vi "Build Tree.vi"(5 "Panel":refnum<vi>, 7 "Tree":refnum<vi>, 9 "Changed Actors":refnum<class "Message Enqueuer.lvclass">[](array[class]), 10 "Monitor Data":refnum<class "Monitor Data.lvclass">) -> (2 "Stopped Actors":string[](array[string]))   [LabVIEW 2023, in "Monitored Actor.lvlib" / "Classic Monitor.lvclass"]
doc: "Manages the tree.\n\nCopyright: MGI 2016\nAuthor: Derek Trepanier"
uses:
  Classic Monitor.lvclass
  Monitor Data/Monitor Data.lvclass
  builds/Framework/Actor Framework.lvlibp/1abvi3w/vi.lib/ActorFramework/Message Enqueuer/Message Enqueuer.lvclass
  Classic Monitor.lvclass/Classic Monitor.ctl
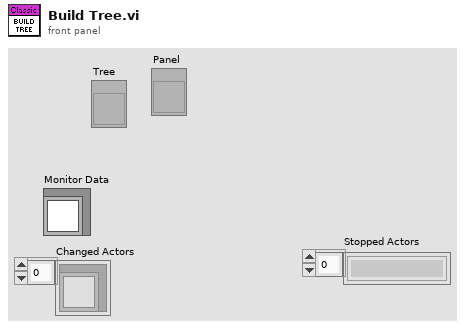
[diagram p1: front panel]
types:
  T1 = typedef "Monitored Actor.lvlib/Monitor Data.lvclass/Actor Data.ctl" = cluster{"Actor Type":string, "Actor Core VI":string, "Self":refnum<class "Message Enqueuer.lvclass">, "Caller":refnum<class "Message Enqueuer.lvclass">, "Actor Label":string, "Last Ping":dbl}
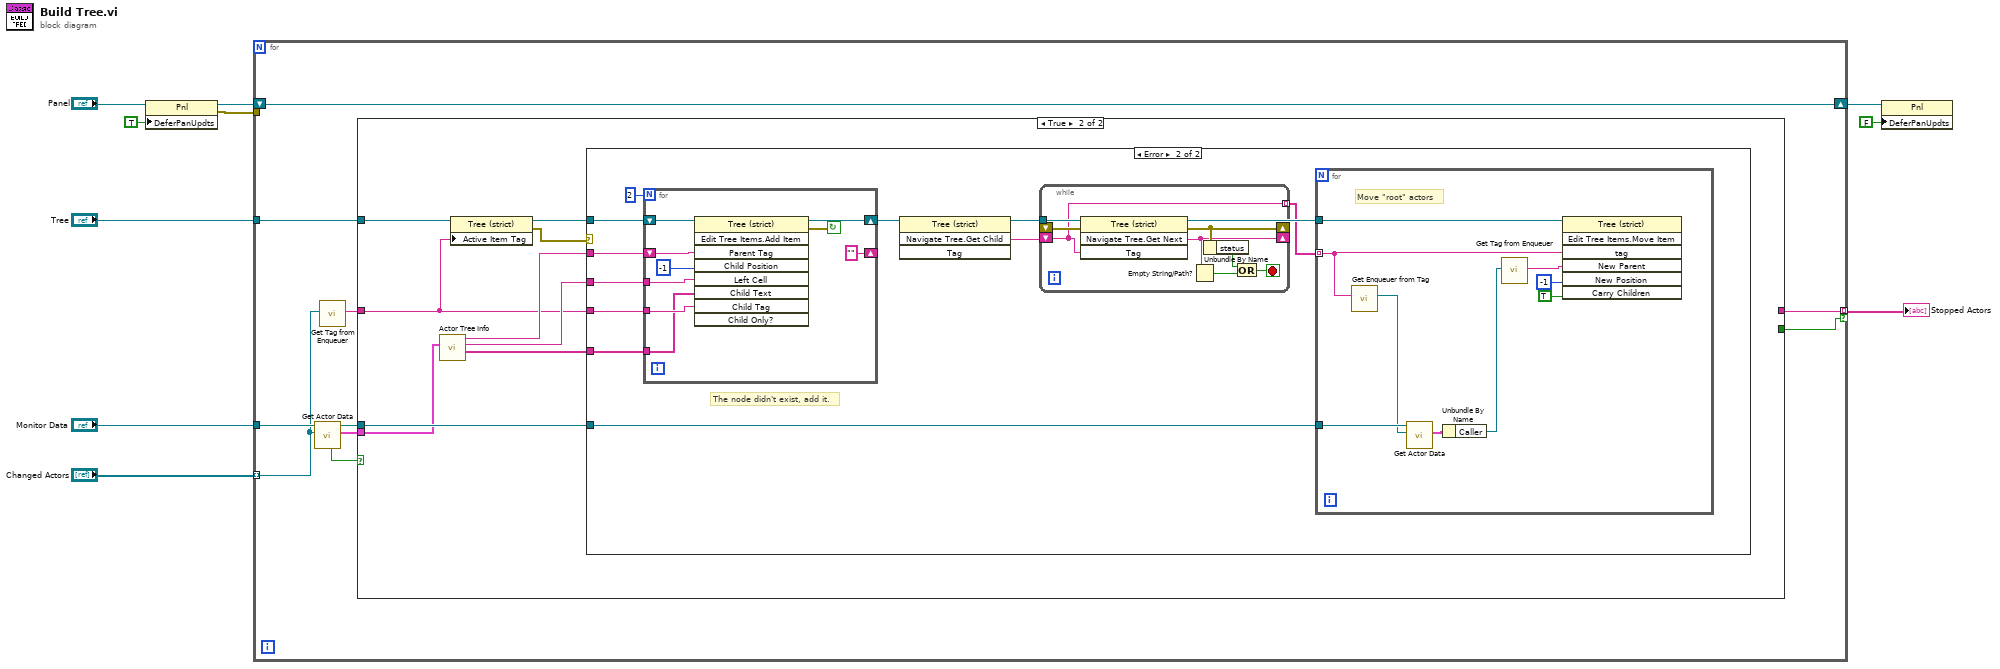
[diagram p0: block diagram]
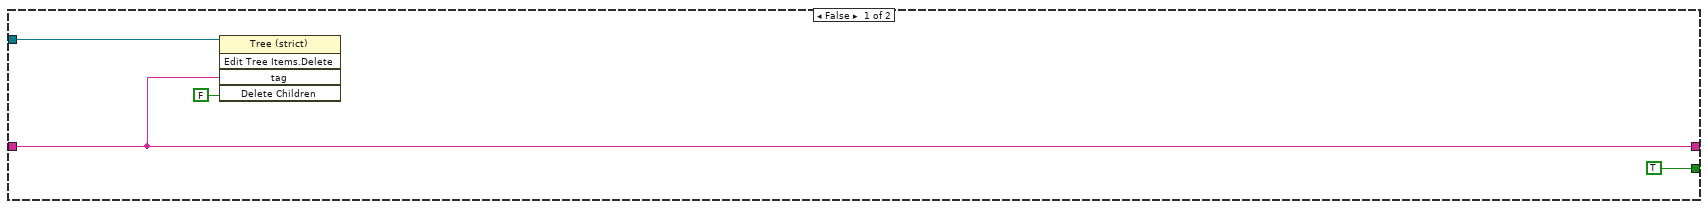
[diagram p2: hidden frame]
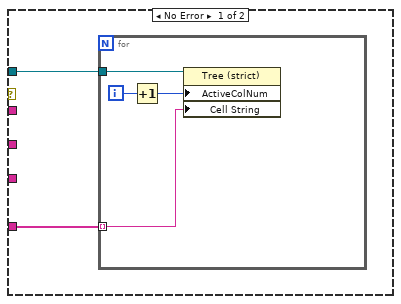
[diagram p3: hidden frame]
diagram:
  n1 = property class="Pnl"(reference="Panel", "DeferPanUpdts"=TRUE ("Defer Panel Updates")) -> (reference out=w5:refnum<vi>, error out=w1:errorcluster)  [unwired: 1 in]
  n2 = for {
    tunnel: "Monitor Data" -> [w18]
    tunnel: "Tree" -> [w20]
    shift-right: [w19] -> w4
    shift-left: w5 -> [w19]
    tunnel: "Changed Actors" -> [w15] mode=indexing
    tunnel: [w12] -> w2 mode=indexing if=w11
    tunnel: w1 -> [_]
    n3 = call "Get Actor Data.vi"("Actor's Self Q"=w15, "Monitor Data in"=w18) -> ("Actor Data"=w16:T1, "Monitor Data out"=w17:refnum<class "Monitor Data.lvclass">, "Found?"=w13:bool)  [unwired: 5 in, 2 out]
    n4 = call "Get Tag from Enqueuer.vi"("Enqueuer"=w15) -> ("Tag"=w14:string)  [unwired: 10 in]
    n5 = case shown="True" w13 {
      tunnel: w20 -> [w24 w33]
      tunnel: w17 -> [_ w28]
      tunnel: w16 -> [_ w27]
      tunnel: w14 -> [w22 w25]
      tunnel: [w22 _] -> w12
      tunnel: [TRUE _] -> w11
      frame False {
        n6 = invoke class="Tree (strict)" method="Edit Tree Items.Delete"(reference=w24, "tag"=w22, "Delete Children"=FALSE ("Delete Children?")) -> ()  [unwired: 2 in, 5 out]
      }
      frame True {
        n7 = call "Actor Tree Info.vi"("Actor Data"=w27) -> ("Column Data"=w30:string[], "Node Name"=w26:string, "Parent Tag"=w29:string)  [unwired: 8 in]
        n8 = property class="Tree (strict)"(reference=w33, "Active Item Tag"=w25) -> (reference out=w31:refnum<vi>, error out=w32:errorcluster)  [unwired: 1 in]
        n9 = case shown="Error" w32 {
          tunnel: w31 -> [w35 w50]
          tunnel: w30 -> [w34 w49]
          tunnel: w29 -> [_ w48]
          tunnel: w28 -> [_ w46]
          tunnel: w26 -> [_ w45]
          tunnel: w25 -> [_ w44]
          frame No Error {
            n10 = for {
              tunnel: w35 -> [w39]
              tunnel: w34 -> [w37] mode=indexing
              i -> [w38]
              n11 = Increment(x=w38) -> (x+1=w36:i32)
              n12 = property class="Tree (strict)"(reference=w39, "ActiveColNum"=w36, "Cell String"=w37) -> ()  [unwired: 1 in, 2 out]
            }
          }
          frame Error {
            # "The node didn't exist, add it."
            n13 = for {
              N: 2 -> [_]
              tunnel: w49 -> [w59]
              shift-right: ["" ("Parent Tag")] -> _
              shift-left: w48 -> [w65]
              shift-right: [w62] -> w43
              shift-left: w50 -> [w67]
              tunnel: w45 -> [w61]
              tunnel: w44 -> [w60]
              stop <- w63 continue-if-true
              n14 = invoke class="Tree (strict)" method="Edit Tree Items.Add Item"(reference=w67, "Parent Tag"=w65, "Child Position"=-1, "Left Cell"=w61, "Child Text"=w59, "Child Tag"=w60) -> (reference out=w62:refnum<vi>, error out=w63:errorcluster)  [unwired: 3 in, 7 out]
            }
            n15 = invoke class="Tree (strict)" method="Navigate Tree.Get Child"(reference=w43) -> (reference out=w42:refnum<vi>, "Navigate Tree:Get Child"=w41:string)  [unwired: 3 in, 2 out]
            n16 = while {
              shift-right: [w52] -> _
              shift-left: w41 -> [w51]
              tunnel: w42 -> [w58]
              shift-right: [w53] -> _
              shift-left: _ -> [w57]
              tunnel: [w51] -> w40 mode=indexing
              stop <- w55 stop-if-true
              n17 = invoke class="Tree (strict)" method="Navigate Tree.Get Next"(reference=w58, error in=w57, "Tag"=w51) -> (error out=w53:errorcluster, "Navigate Tree:Get Next Item"=w52:string)  [unwired: 1 in, 2 out]
              n18 = Empty String/Path?(string/path=w52) -> (empty?=w56:bool)
              n19 = Unbundle By Name(w53) -> ("status"=w54:bool)
              n20 = Compound Arithmetic op=OR(w54, w56) -> (w55:bool)
            }
            n21 = for {
              tunnel: w46 -> [w76]
              tunnel: w42 -> [w73]
              tunnel: w40 -> [w68] mode=indexing
              # "Move \"root\" actors"
              n22 = call "Get Enqueuer from Tag.vi"("Tag"=w68) -> ("Enqueuer"=w75:refnum<class "Message Enqueuer.lvclass">)  [unwired: 10 in]
              n23 = call "Get Actor Data.vi"("Actor's Self Q"=w75, "Monitor Data in"=w76) -> ("Actor Data"=w74:T1)  [unwired: 5 in, 4 out]
              n24 = Unbundle By Name(w74) -> ("Caller"=w72:refnum<class "Message Enqueuer.lvclass">)
              n25 = call "Get Tag from Enqueuer.vi"("Enqueuer"=w72) -> ("Tag"=w71:string)  [unwired: 10 in]
              n26 = invoke class="Tree (strict)" method="Edit Tree Items.Move Item"(reference=w73, "tag"=w68, "New Parent"=w71, "New Position"=-1, "Carry Children"=TRUE ("Carry Children?")) -> ()  [unwired: 2 in, 7 out]
            }
          }
        }
      }
    }
  }
  "Stopped Actors" <- w2
  n27 = property class="Pnl"(reference=w4, "DeferPanUpdts"=FALSE ("Defer Panel Updates")) -> ()  [unwired: 1 in, 2 out]
